vi "Start Administrator Console.vi"(8 "error in (no error)":errorcluster, 11 "Message Queues":T1) -> (0 "error out":errorcluster, 3 "Administrator Console Reference":refnum<vi>)   [LabVIEW 2024]
doc: "Starts the Administrator Console."
uses:
  Shared/Message Queue/Server Message Queues.ctl
  Shared/Message Queue/Message Cluster.ctl
  Shared/Message Queue.lvlib
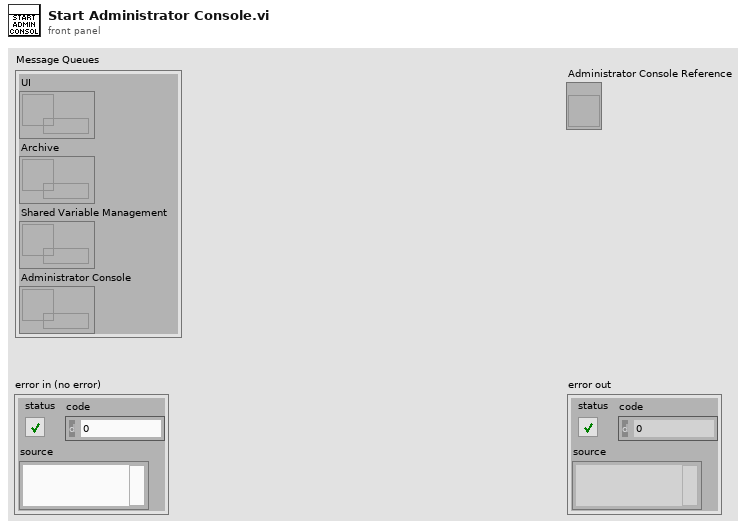
[diagram p1: front panel]
types:
  T1 = typedef "Message Queue.lvlib/Server Message Queues.ctl" = cluster{"UI":refnum<queue>, "Archive":refnum<queue>, "Shared Variable Management":refnum<queue>, "Administrator Console":refnum<queue>}
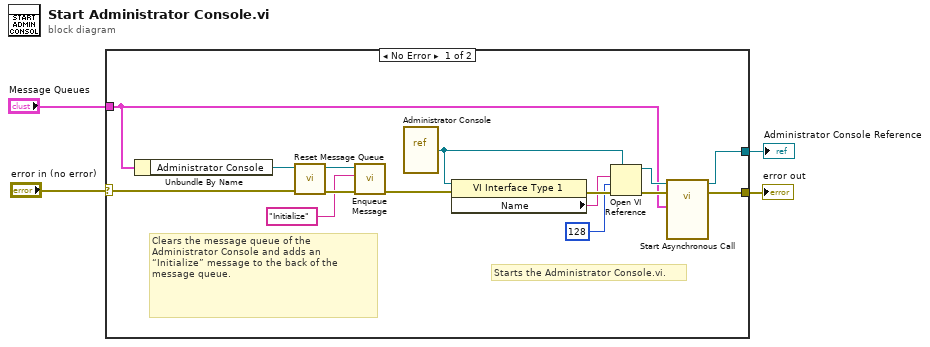
[diagram p0: block diagram]
diagram:
  n1 = case shown="No Error" "error in (no error)" {
    selector: "error in (no error)" -> [w5 w20]
    tunnel: [w9 w20] -> w4
    tunnel: [w8 _] -> w3
    tunnel: "Message Queues" -> [w6 _]
    frame No Error {
      # "Clears the message queue of the Administrator Console and adds an “Initialize” message to the back of the message queue."
      # "Starts the Administrator Console.vi."
      n2 = Unbundle By Name(w6) -> ("Administrator Console"=w17:refnum<queue>)
      n3 = call "Reset Message Queue.vi"("error in (no error)"=w5, "Message Queue"=w17) -> ("error out"=w19:errorcluster, "dup Message Queue"=w18:refnum<queue>)  [unwired: 8 in]
      n4 = call "Enqueue Message.vi"("error in (no error)"=w19, "Message"="Initialize", "Message Queue"=w18) -> ("error out"=w7:errorcluster)  [unwired: 7 in, 1 out]
      n5 = vi-ref "Administrator Console.vi"() -> (w11:refnum<vi>)
      n6 = property class="VI Interface Type 1"(reference=w11, error in=w7) -> (error out=w15:errorcluster, "Name"=w12:string)  [unwired: 1 out]
      n7 = Open VI Reference(type specifier VI Refnum (for type only)=w11, vi path=w12, options=128, error in (no error)=w15) -> (vi reference=w10:refnum<vi>, error out=w14:errorcluster)  [unwired: 2 in]
      n8 = call-by-ref "Start Asynchronous Call"(reference=w10, error in=w14, "Message Queues"=w6) -> (reference out=w8:refnum<vi>, error out=w9:errorcluster)  [unwired: 10 in, 1 out]
    }
    frame Error {
    }
  }
  "error out" <- w4
  "Administrator Console Reference" <- w3
